vi "SaveConfigPhospho.vi"(0 "configuration file path":path caption="chemin du fichier de configuration", 1 "Associated files":T1, 2 "Pulse properties":T3={"N pulses"=0, "Samples"=0, "Last samples"=0, "AO pulse ticks"=0, "Skip samples"=0, "N samples/decay"=0, "Sliding Step \n(nb pulses)"=0, "Slidiing window\n (nb pulses)"=0, "Interpoints \ninterval (ms)"=100.0, "Repeat \neach point"=8, "Number of points"=0, "Mean and Time-Lapsed on Point Number"=0, "Oxygen dye type"=10106, "N samples/ decay min"=0, "Interpulse Interval"=0.0, "Wait"=30} {"Oxygen dye type" items=["PtP-C343 (30 kDa)", "PtP-C343 (65 KDa)"]; "Repeat \neach point" min=2 step=1}, 3 "Acquisition properties":T2) -> ()   [LabVIEW 2013, in "Phosphorescence - Mode.lvlib"]
uses:
  Phosphorescence - Mode.lvlib
  <vilib>/Utility/config.llb/Write Key (I32).vi
  <vilib>/Utility/config.llb/Write Key (String).vi
  <vilib>/Utility/config.llb/Write Key (Double).vi
  <vilib>/Utility/config.llb/NI_LVConfig.lvlib
  File management.lvlib
panel:
  in  "Wait":i32
  out "TDMS path":string
  out "Interpulse Interval":dbl
  out "N samples/ decay min":i32
  in  "Synchro":bool
  out "Oxygen dye type":i16(ring)=10106 items=["PtP-C343 (30 kDa)", "PtP-C343 (65 KDa)"]
  out "Results file":string
  out "Timing file":string
  out "Raw images file":string[][](array[string])
  in  "Point Number":i32
  in  "Repeat \neach point":i32=8 min=2 step=1
  in  "Interpoints \ninterval (ms)":dbl=100.0
  in  "Number of points":i32
  out "Reference text file":string
  out "Reference image files":string[](array[string])
  out "Mean and fit file":string
  in  "Selection coordinates":dbl[](array[numeric])=[0.5875, 0.6937500000000001, 0.9437500000000001, 0.9750000000000001, 0.5875, 0.7364583333333334, 0.5916666666666667, 0.696875, 0.9333333333333333, 0.6937500000000001, 0.9437500000000001, 0.7208333333333333, 0.7822916666666666, 0.9750000000000001, 0.7562500000000001, 0.971875, 0.5875, 0.7364583333333334]
  in  "Pictures coordinates":dbl[](array[numeric])=[0.5875, 0.6937500000000001, 0.9437500000000001, 0.9750000000000001, 0.5875, 0.7364583333333334, 0.5916666666666667, 0.696875, 0.9333333333333333, 0.6937500000000001, 0.9437500000000001, 0.7208333333333333, 0.7822916666666666, 0.9750000000000001, 0.7562500000000001, 0.971875, 0.5875, 0.7364583333333334]
  in  "pwr_rel":dbl(slide)=0.01 min=0.01 max=1.0 step=0.005 scale=0.01..1.0 scale format="%.2f"
  in  "Channel Acq":i32 min=0 max=1 step=1
  in  "scan rate (kHz)":dbl=1000.0 caption="Rate (kHz)"
  in  "Last samples":i32=5
  in  "Sliding Step \n(nb pulses)":i32=8 min=2 step=1
  in  "Slidiing window\n (nb pulses)":i32=8 min=2 step=1
  in  "Skip samples":i32=12
  in  "Samples":i32=1500 caption="Total scans"
  in  "N samples/decay":i32=150
  in  "pulse ticks":i32=8 min=2 step=1
  in  "N pulses":i32=10
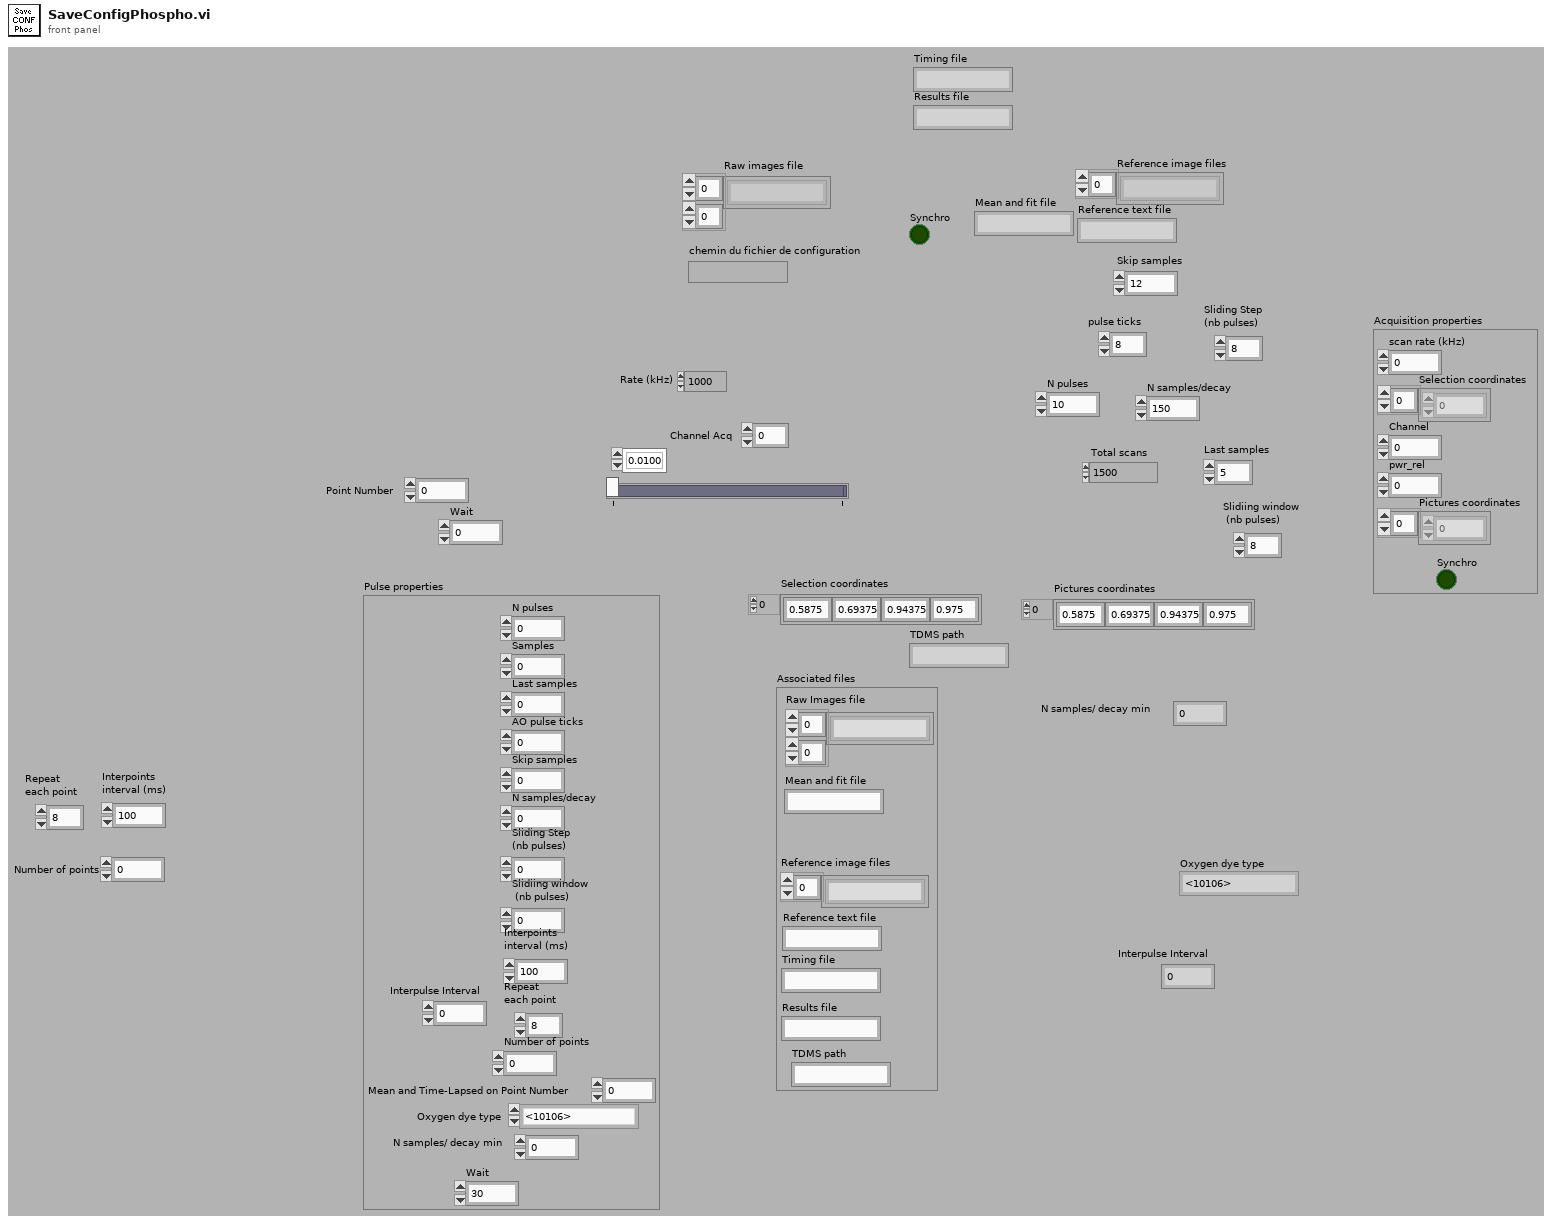
[diagram p1: front panel]
types:
  T1 = cluster{"Raw Images file":string[][], "Mean and fit file":string, "Reference image files":string[], "Reference text file":string, "Timing file":string, "Results file":string, "TDMS path":string}
  T2 = cluster{"scan rate (kHz)":dbl, "Selection coordinates":dbl[], "Channel":i32, "pwr_rel":dbl, "Pictures coordinates":dbl[], "Synchro":bool}
  T3 = cluster{"N pulses":i32, "Samples":i32, "Last samples":i32, "AO pulse ticks":i32, "Skip samples":i32, "N samples/decay":i32, "Sliding Step \n(nb pulses)":i32, "Slidiing window\n (nb pulses)":i32, "Interpoints \ninterval (ms)":dbl, "Repeat \neach point":i32, "Number of points":i32, "Mean and Time-Lapsed on Point Number":i32, "Oxygen dye type":i16, "N samples/ decay min":i32, "Interpulse Interval":dbl, "Wait":i32}
  T4 = enum16{"fractional", "engineering", "exponential"}
  T5 = typedef "NI_LVConfig.lvlib/Config Data RefNum.ctl" = refnum<k1>
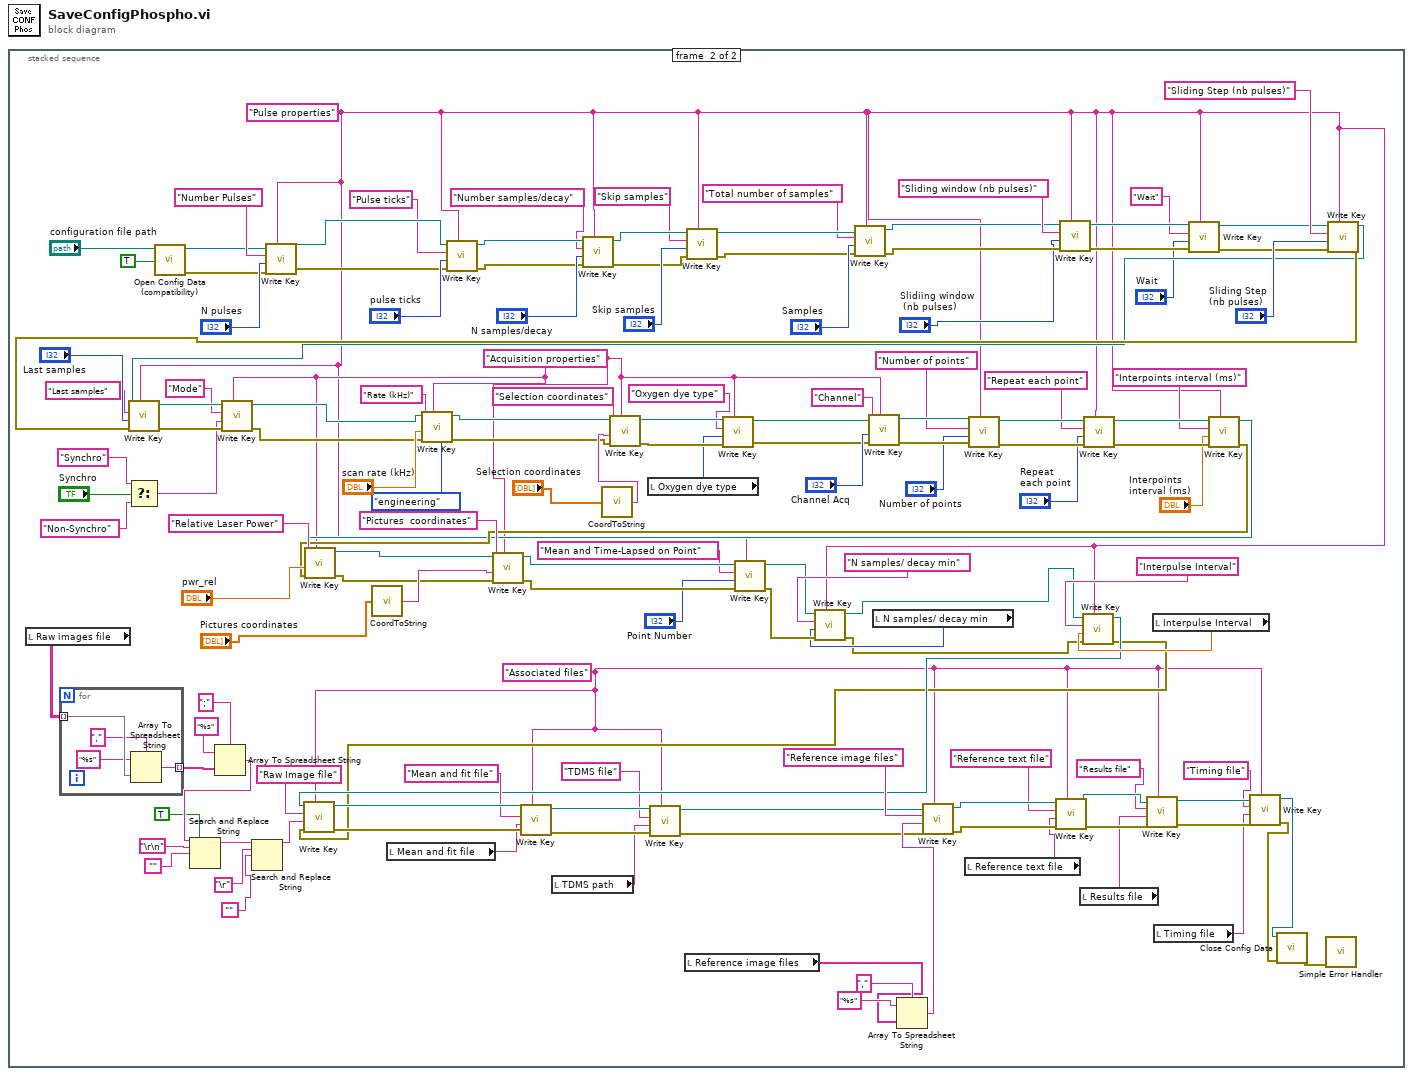
[diagram p0: block diagram]
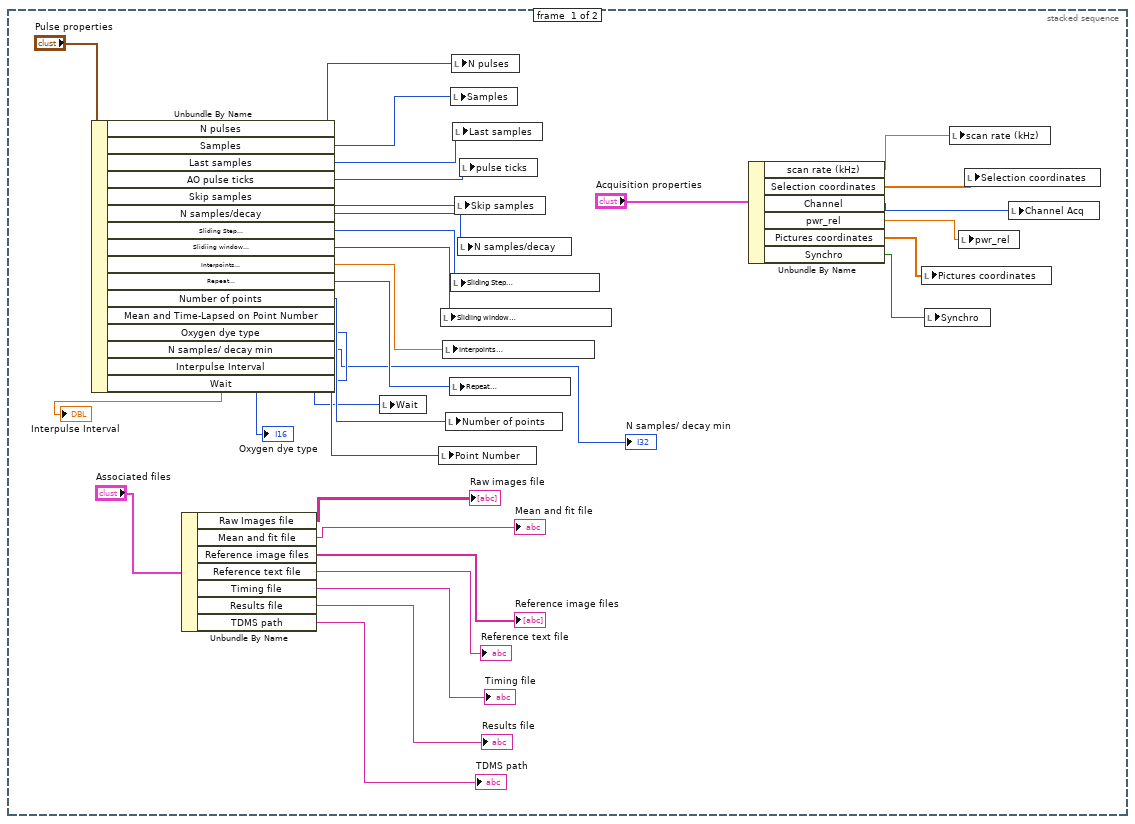
[diagram p2: hidden frame]
diagram:
  n1 = stacked-sequence {
    frame #0 {
      n2 = Unbundle By Name ("Désassembler par nom")("Pulse properties") -> ("N pulses"=w31:i32, "Samples"=w30:i32, "Last samples"=w29:i32, "AO pulse ticks"=w28:i32, "Skip samples"=w27:i32, "N samples/decay"=w26:i32, "Sliding Step \n(nb pulses)"=w25:i32, "Slidiing window\n (nb pulses)"=w24:i32, "Interpoints \ninterval (ms)"=w13:dbl, "Repeat \neach point"=w12:i32, "Number of points"=w11:i32, "Mean and Time-Lapsed on Point Number"=w10:i32, "Oxygen dye type"=→"Oxygen dye type":i16, "N samples/ decay min"=→"N samples/ decay min":i32, "Interpulse Interval"=→"Interpulse Interval":dbl, "Wait"=w1:i32)
      n3 = Unbundle By Name("Associated files") -> ("Raw Images file"=→"Raw images file":string[][], "Mean and fit file"=→"Mean and fit file":string, "Reference image files"=→"Reference image files":string[], "Reference text file"=→"Reference text file":string, "Timing file"=→"Timing file":string, "Results file"=→"Results file":string, "TDMS path"=→"TDMS path":string)
      n4 = local write "Wait"(w1) -> ()
      n5 = local write "Point Number"(w10) -> ()
      n6 = local write "Slidiing window\n (nb pulses)"(w24) -> ()
      n7 = local write "Interpoints \ninterval (ms)"(w13) -> ()
      n8 = local write "Number of points"(w11) -> ()
      n9 = local write "Repeat \neach point"(w12) -> ()
      n10 = local write "Samples"(w30) -> ()
      n11 = local write "Sliding Step \n(nb pulses)"(w25) -> ()
      n12 = local write "N pulses"(w31) -> ()
      n13 = local write "Last samples"(w29) -> ()
      n14 = local write "Skip samples"(w27) -> ()
      n15 = local write "N samples/decay"(w26) -> ()
      n16 = local write "pulse ticks"(w28) -> ()
      n17 = Unbundle By Name("Acquisition properties") -> ("scan rate (kHz)"=w22:dbl, "Selection coordinates"=w18:dbl[], "Channel"=w20:i32, "pwr_rel"=w21:dbl, "Pictures coordinates"=w19:dbl[], "Synchro"=w5:bool)
      n18 = local write "Pictures coordinates"(w19) -> ()
      n19 = local write "Synchro"(w5) -> ()
      n20 = local write "scan rate (kHz)"(w22) -> ()
      n21 = local write "pwr_rel"(w21) -> ()
      n22 = local write "Selection coordinates"(w18) -> ()
      n23 = local write "Channel Acq"(w20) -> ()
    }
    frame #1 {
      w40 = "Associated files" ("key")
      w58 = "Acquisition properties" ("section")
      w34 = "Pulse properties" ("section")
      n24 = local read "Raw images file"() -> (w94:string[][])
      n25 = for {
        tunnel: w94 -> [w180] mode=indexing
        tunnel: [w177] -> w83 mode=indexing
        n26 = Array To Spreadsheet String(delimiter (Tab)="," ("séparateur (Tabulation)"), array=w180, 3:"%s" ("chaîne de format")) -> (spreadsheet string=w177:string)
      }
      n27 = Select(t="Synchro" ("key"), s="Synchro", f="Non-Synchro" ("key")) -> (s? t:f=w60:string)
      n28 = call <vilib>:"Open Config Data (compatibility).vi"("create file if necessary (T)"=TRUE ("create file if necessary? (T)"), "configuration file path"="configuration file path") -> ("error out"=w135:errorcluster, "refnum"=w134:T5)  [unwired: 7 in, 1 out]
      n29 = Array To Spreadsheet String(delimiter (Tab)=";" ("séparateur (Tabulation)"), array=w83, 3:"%s" ("chaîne de format")) -> (spreadsheet string=w80:string)
      n30 = Search and Replace String(replace all?=TRUE ("tout remplacer ? (F)"), input string=w80, search string="\r\n", replace string="") -> (result string=w76:string)  [unwired: 1 in, 6 out]
      n31 = Search and Replace String(input string=w76, search string="\r", replace string="") -> (result string=w73:string)  [unwired: 1 in, 7 out]
      n32 = call-poly <vilib>:"Write Key.vi"("section"=w34, "error in (no error)"=w135, "value"="N pulses", "key"="Number Pulses", "refnum"=w134) -> ("error out"=w146:errorcluster, "refnum out"=w141:T5)  [unwired: 5 out]
      n33 = call "CoordToString.vi"("coordinates"="Pictures coordinates") -> ("String coordinates"=w176:string)
      n34 = local read "Mean and fit file"() -> (w118:string)
      n35 = call-poly <vilib>:"Write Key.vi"("section"=w34, "error in (no error)"=w146, "value"="pulse ticks", "key"="Pulse ticks", "refnum"=w141) -> ("error out"=w145:errorcluster, "refnum out"=w140:T5)  [unwired: 5 out]
      n36 = local read "TDMS path"() -> (w42:string)
      n37 = call-poly <vilib>:"Write Key.vi"("section"=w34, "error in (no error)"=w145, "value"="N samples/decay", "key"="Number samples/decay", "refnum"=w140) -> ("error out"=w144:errorcluster, "refnum out"=w143:T5)  [unwired: 5 out]
      n38 = call "CoordToString.vi"("coordinates"="Selection coordinates") -> ("String coordinates"=w174:string)
      n39 = local read "Oxygen dye type"() -> (w68:i16)
      n40 = local read "Reference image files"() -> (w114:string[])
      n41 = call-poly <vilib>:"Write Key.vi"("section"=w34, "error in (no error)"=w144, "value"="Skip samples", "key"="Skip samples", "refnum"=w143) -> ("error out"=w152:errorcluster, "refnum out"=w151:T5)  [unwired: 5 out]
      n42 = call-poly <vilib>:"Write Key.vi"("section"=w34, "error in (no error)"=w152, "value"="Samples", "key"="Total number of samples", "refnum"=w151) -> ("error out"=w129:errorcluster, "refnum out"=w130:T5)  [unwired: 5 out]
      n43 = local read "N samples/ decay min"() -> (w54:i32)
      n44 = Array To Spreadsheet String(delimiter (Tab)="," ("séparateur (Tabulation)"), array=w114, 3:"%s" ("chaîne de format")) -> (spreadsheet string=w113:string)
      n45 = local read "Reference text file"() -> (w117:string)
      n46 = call-poly <vilib>:"Write Key.vi"("section"=w34, "error in (no error)"=w129, "value"="Slidiing window\n (nb pulses)", "key"="Sliding window (nb pulses)", "refnum"=w130) -> ("error out"=w37:errorcluster, "refnum out"=w39:T5)  [unwired: 5 out]
      n47 = local read "Results file"() -> (w86:string)
      n48 = local read "Interpulse Interval"() -> (w52:dbl)
      n49 = local read "Timing file"() -> (w87:string)
      n50 = call-poly <vilib>:"Write Key.vi"("section"=w34, "error in (no error)"=w37, "value"="Wait", "key"="Wait", "refnum"=w39) -> ("error out"=w36:errorcluster, "refnum out"=w38:T5)  [unwired: 5 out]
      n51 = call-poly <vilib>:"Write Key.vi"("section"=w34, "error in (no error)"=w36, "value"="Sliding Step \n(nb pulses)", "key"="Sliding Step (nb pulses)", "refnum"=w38) -> ("error out"=w160:errorcluster, "refnum out"=w159:T5)  [unwired: 5 out]
      n52 = call-poly <vilib>:"Write Key.vi"("section"=w34, "error in (no error)"=w160, "value"="Last samples", "key"="Last samples", "refnum"=w159) -> ("error out"=w64:errorcluster, "refnum out"=w66:T5)  [unwired: 5 out]
      n53 = call-poly <vilib>:"Write Key.vi"("section"=w58, "error in (no error)"=w64, "value"=w60, "key"="Mode", "refnum"=w66) -> ("error out"=w63:errorcluster, "refnum out"=w65:T5)  [unwired: 1 in, 4 out]
      n54 = call-poly <vilib>:"Write Key.vi"("format (fractional)"=T4."engineering", "section"=w58, "error in (no error)"=w63, "value"="scan rate (kHz)", "key"="Rate (kHz)", "refnum"=w65) -> ("error out"=w162:errorcluster, "refnum out"=w149:T5)  [unwired: 2 in, 2 out]
      n55 = call-poly <vilib>:"Write Key.vi"("section"=w58, "error in (no error)"=w162, "value"=w174, "key"="Selection coordinates", "refnum"=w149) -> ("error out"=w69:errorcluster, "refnum out"=w72:T5)  [unwired: 1 in, 4 out]
      n56 = call-poly <vilib>:"Write Key.vi"("section"=w58, "error in (no error)"=w69, "value"=w68, "key"="Oxygen dye type", "refnum"=w72) -> ("error out"=w70:errorcluster, "refnum out"=w71:T5)  [unwired: 5 out]
      n57 = call-poly <vilib>:"Write Key.vi"("section"=w58, "error in (no error)"=w70, "value"="Channel Acq", "key"="Channel", "refnum"=w71) -> ("error out"=w112:errorcluster, "refnum out"=w109:T5)  [unwired: 5 out]
      n58 = call-poly <vilib>:"Write Key.vi"("section"=w34, "error in (no error)"=w112, "value"="Number of points", "key"="Number of points", "refnum"=w109) -> ("error out"=w111:errorcluster, "refnum out"=w105:T5)  [unwired: 1 in, 4 out]
      n59 = call-poly <vilib>:"Write Key.vi"("section"=w34, "error in (no error)"=w111, "value"="Repeat \neach point", "key"="Repeat each point", "refnum"=w105) -> ("error out"=w110:errorcluster, "refnum out"=w106:T5)  [unwired: 5 out]
      n60 = call-poly <vilib>:"Write Key.vi"("section"=w34, "error in (no error)"=w110, "value"="Interpoints \ninterval (ms)", "key"="Interpoints interval (ms)", "refnum"=w106) -> ("error out"=w108:errorcluster, "refnum out"=w107:T5)  [unwired: 3 in, 2 out]
      n61 = call-poly <vilib>:"Write Key.vi"("section"=w58, "error in (no error)"=w108, "value"="pwr_rel", "key"="Relative Laser Power", "refnum"=w107) -> ("error out"=w157:errorcluster, "refnum out"=w156:T5)  [unwired: 3 in, 2 out]
      n62 = call-poly <vilib>:"Write Key.vi"("section"=w58, "error in (no error)"=w157, "value"=w176, "key"="Pictures  coordinates", "refnum"=w156) -> ("error out"=w97:errorcluster, "refnum out"=w98:T5)  [unwired: 1 in, 4 out]
      n63 = call-poly <vilib>:"Write Key.vi"("section"=w34, "error in (no error)"=w97, "value"="Point Number", "key"="Mean and Time-Lapsed on Point", "refnum"=w98) -> ("error out"=w56:errorcluster, "refnum out"=w53:T5)  [unwired: 5 out]
      n64 = call-poly <vilib>:"Write Key.vi"("section"=w34, "error in (no error)"=w56, "value"=w54, "key"="N samples/ decay min", "refnum"=w53) -> ("error out"=w48:errorcluster, "refnum out"=w50:T5)  [unwired: 5 out]
      n65 = call-poly <vilib>:"Write Key.vi"("section"=w34, "error in (no error)"=w48, "value"=w52, "key"="Interpulse Interval", "refnum"=w50) -> ("error out"=w47:errorcluster, "refnum out"=w49:T5)  [unwired: 3 in, 2 out]
      n66 = call-poly <vilib>:"Write Key.vi"("section"=w40, "error in (no error)"=w47, "value"=w73, "key"="Raw Image file", "refnum"=w49) -> ("error out"=w124:errorcluster, "refnum out"=w126:T5)  [unwired: 1 in, 4 out]
      n67 = call-poly <vilib>:"Write Key.vi"("section"=w40, "error in (no error)"=w124, "value"=w118, "key"="Mean and fit file", "refnum"=w126) -> ("error out"=w46:errorcluster, "refnum out"=w44:T5)  [unwired: 1 in, 4 out]
      n68 = call-poly <vilib>:"Write Key.vi"("section"=w40, "error in (no error)"=w46, "value"=w42, "key"="TDMS file", "refnum"=w44) -> ("error out"=w45:errorcluster, "refnum out"=w43:T5)  [unwired: 1 in, 4 out]
      n69 = call-poly <vilib>:"Write Key.vi"("section"=w40, "error in (no error)"=w45, "value"=w113, "key"="Reference image files", "refnum"=w43) -> ("error out"=w123:errorcluster, "refnum out"=w125:T5)  [unwired: 1 in, 4 out]
      n70 = call-poly <vilib>:"Write Key.vi"("section"=w40, "error in (no error)"=w123, "value"=w117, "key"="Reference text file", "refnum"=w125) -> ("error out"=w90:errorcluster, "refnum out"=w93:T5)  [unwired: 1 in, 4 out]
      n71 = call-poly <vilib>:"Write Key.vi"("section"=w40, "error in (no error)"=w90, "value"=w86, "key"="Results file", "refnum"=w93) -> ("error out"=w89:errorcluster, "refnum out"=w92:T5)  [unwired: 1 in, 4 out]
      n72 = call-poly <vilib>:"Write Key.vi"("section"=w40, "error in (no error)"=w89, "value"=w87, "key"="Timing file", "refnum"=w92) -> ("error out"=w88:errorcluster, "refnum out"=w91:T5)  [unwired: 1 in, 4 out]
      n73 = call <vilib>:"Close Config Data.vi"("error in (no error)"=w88, "refnum"=w91) -> ("error out"=w161:errorcluster)  [unwired: 1 in, 8 out]
      n74 = call <vilib>:"Simple Error Handler.vi"("error in (no error)"=w161) -> ()  [unwired: 1 in, 8 out]
    }
  }
